vi "navX Example v2 - Dual navX.vi"() -> ()   [LabVIEW 2015]
uses:
  navX Library v2/TypeDefs/Flags/Z900_navX_Flags_OpStatusTypeDef.ctl
  navX Library v2/TypeDefs/Flags/Z900_navX_Flags_CalibrationStatusTypeDef.ctl
  navX Library v2/TypeDefs/Flags/Z900_navX_Flags_HardwareRevTypeDef.ctl
  navX Library v2/TypeDefs/Flags/Z900_navX_Flags_OmnimountConfigTypeDef.ctl
  <vilib>/Rock Robotics/SystemInterfaces/spilib/spi_bus.ctl
  NI WPI/WPI_SerialPort_USB.ctl
  navX Library v2/TypeDefs/Z900_navX_SerialStreamTypeDef.ctl
  navX Library v2/IO/Open/Z900_navX_Open_Serial.vi
  navX Library v2/IO/Open/Z900_navX_Open_SPI.vi
  navX Library v2/navX Library v2.lvlib
  NI WPI/NI WPI Serial USB.lvlib
panel:
  out "Internal error out 2":errorcluster
  out "Internal error out":errorcluster
  in  "stop":bool
  in  "Zero Yaw":bool
  out "YRPHfH 2":T1
  out "Board Information 2":T4 {"Board"."Hardware Revision" items=["navX-MXP"=33, "navX-Micro"=40]; "Omnimount Config" items=["DEFAULT", "X_UP", "X_DOWN", "Y_UP", "Y_DOWN", "Z_UP", "Z_DOWN"]}
  out "Connected 2":bool
  out "Status 2":T7 {"OP Status" items=["INITIALIZING", "SELFTEST_IN_PROGRESS", "ERROR", "IMU_AUTOCAL_IN_PROGRESS", "NORMAL"]; "Calibration Status" items=["IMU_CAL_STATE_MASK"=3, "IMU_CAL_STATE_INPROGRESS"=0, "IMU_CAL_STATE_ACCUMULATE"=1, "IMU_CAL_STATE_COMPLETE"=2]}
  out "YRPHfH":T1
  out "Board Information":T4 {"Board"."Hardware Revision" items=["navX-MXP"=33, "navX-Micro"=40]; "Omnimount Config" items=["DEFAULT", "X_UP", "X_DOWN", "Y_UP", "Y_DOWN", "Z_UP", "Z_DOWN"]}
  out "Connected":bool
  out "Status":T7 {"OP Status" items=["INITIALIZING", "SELFTEST_IN_PROGRESS", "ERROR", "IMU_AUTOCAL_IN_PROGRESS", "NORMAL"]; "Calibration Status" items=["IMU_CAL_STATE_MASK"=3, "IMU_CAL_STATE_INPROGRESS"=0, "IMU_CAL_STATE_ACCUMULATE"=1, "IMU_CAL_STATE_COMPLETE"=2]}
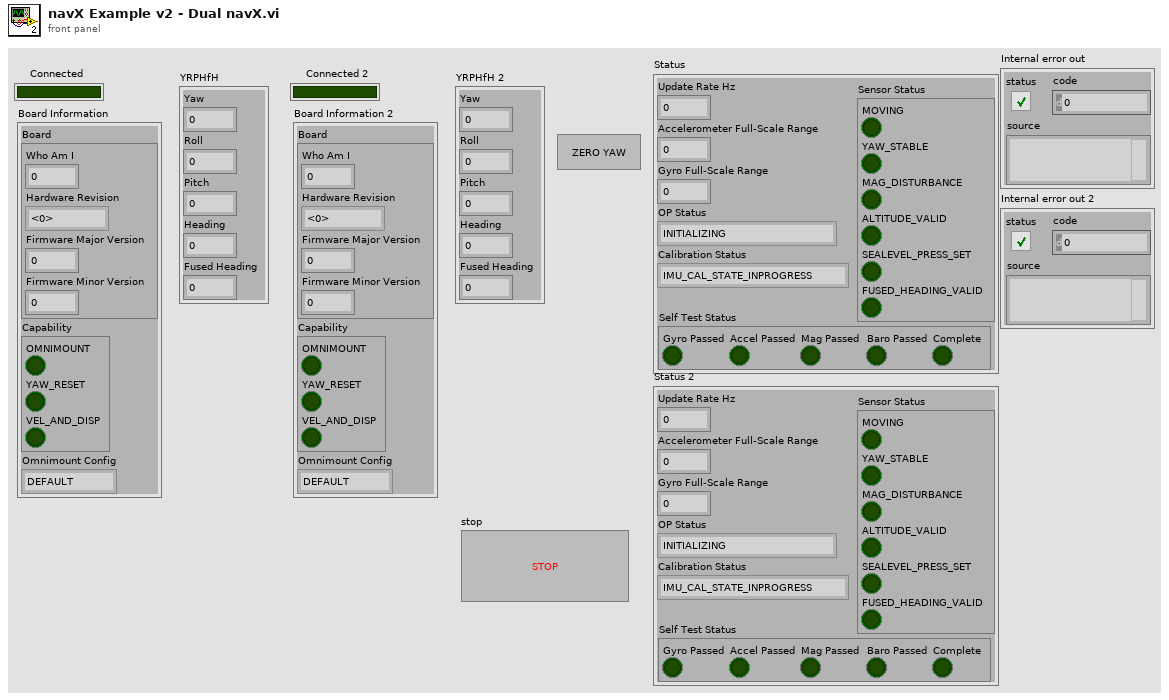
[diagram p1: front panel]
types:
  T1 = cluster{"Yaw":dbl, "Roll":dbl, "Pitch":dbl, "Heading":dbl, "Fused Heading":dbl}
  T2 = typedef "navX Library v2.lvlib/Z900_navX_Flags_HardwareRevTypeDef.ctl" = u8
  T3 = typedef "navX Library v2.lvlib/Z900_navX_Flags_OmnimountConfigTypeDef.ctl" = u8
  T4 = cluster{"Board":cluster{"Who Am I":u8, "Hardware Revision":T2, "Firmware Major Version":u8, "Firmware Minor Version":u8}, "Capability":cluster{"OMNIMOUNT":bool, "YAW_RESET":bool, "VEL_AND_DISP":bool}, "Omnimount Config":T3}
  T5 = typedef "navX Library v2.lvlib/Z900_navX_Flags_OpStatusTypeDef.ctl" = u8
  T6 = typedef "navX Library v2.lvlib/Z900_navX_Flags_CalibrationStatusTypeDef.ctl" = u8
  T7 = cluster{"Update Rate Hz":u8, "Accelerometer Full-Scale Range":u8, "Gyro Full-Scale Range":u16, "OP Status":T5, "Calibration Status":T6, "Sensor Status":cluster{"MOVING":bool, "YAW_STABLE":bool, "MAG_DISTURBANCE":bool, "ALTITUDE_VALID":bool, "SEALEVEL_PRESS_SET":bool, "FUSED_HEADING_VALID":bool}, "Self Test Status":cluster{"Gyro Passed":bool, "Accel Passed":bool, "Mag Passed":bool, "Baro Passed":bool, "Complete":bool}}
  T8 = typedef "navX Library v2.lvlib/Z900_navX_SerialStreamTypeDef.ctl" = enum16{"YRPH", "Quaterinons", "Gyro/Raw", "AHRS", "AHRSAndPositioning"}
  T9 = typedef "NI WPI Serial USB.lvlib/WPI_SerialPort_USB.ctl" = enum16{"Onboard RS-232", "MXP TTL", "USB"}
  T10 = typedef "spi_bus.ctl" = enum16{"SPI On-Board, CS0", "SPI On-Board, CS1", "SPI On-Board, CS2", "SPI On-Board, CS3", "SPI MXP", "Invalid"}
  T11 = typedef "navX Library v2.lvlib/Z900_navX_DeviceTypeDef.ctl" = cluster{"Interface":cluster{"Protocol":T12, "Update Rate (4Hz-60Hz)":u8, "navX Open TypeDef":variant}, "Notify Packet":refnum<notifier>, "Loop VI Refnum":refnum<vi>, "Ready to Close Occurrence Refnum":refnum<k4>}
  T12 = typedef "navX Library v2.lvlib/Z900_navX_ProtocolTypeDef.ctl" = enum16{"SERIAL", "I2C", "SPI"}
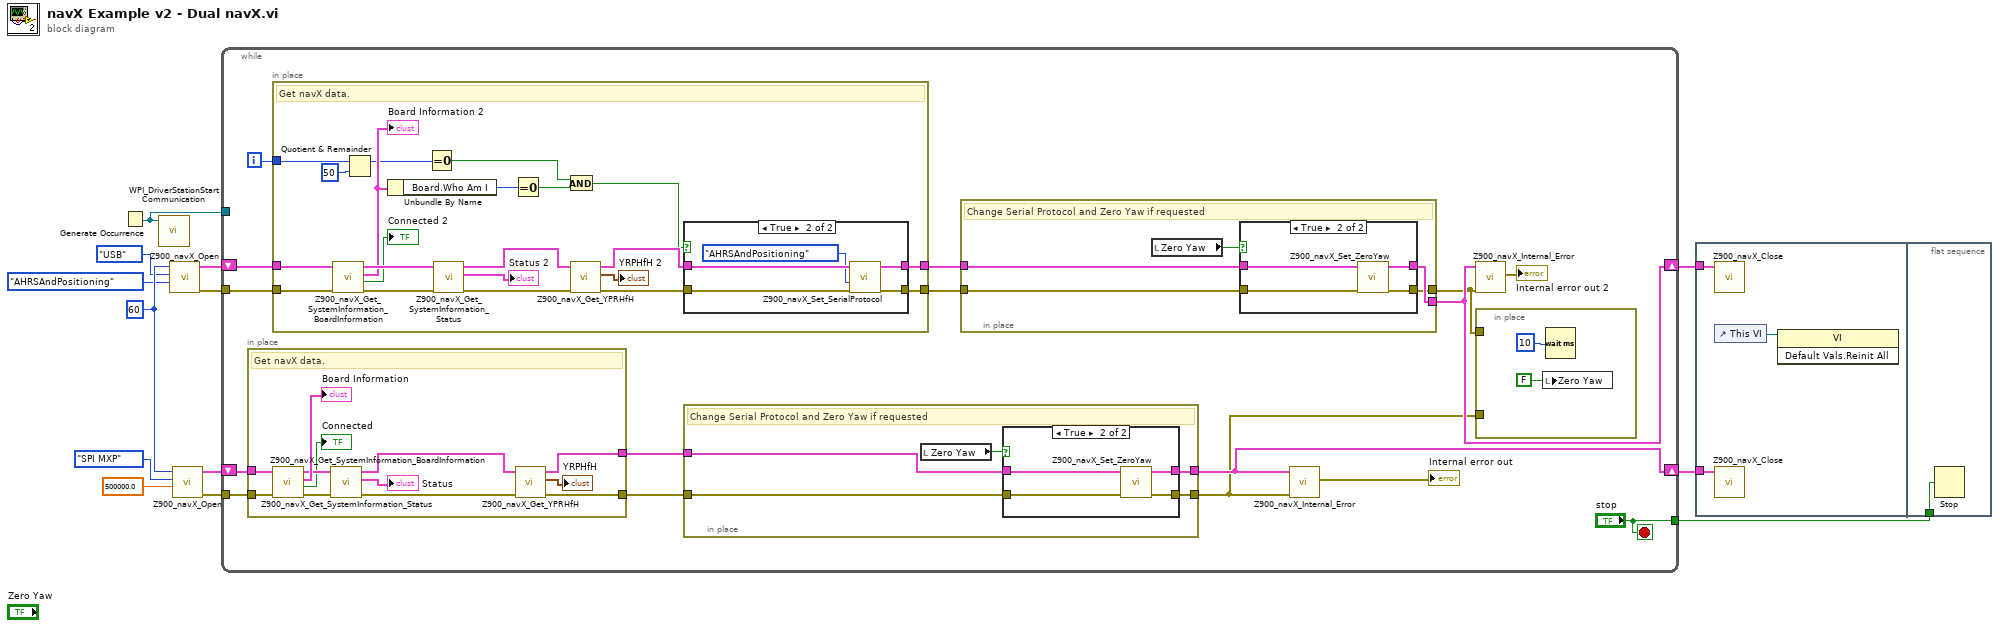
[diagram p0: block diagram]
diagram:
  w9 = u8 60 ("Update Rate (4Hz-60Hz)")
  n1 = Generate Occurrence() -> (w13:refnum<k4>)
  n2 = call <vilib>:"WPI_DriverStationStart Communication.vi"("occurrence"=w13) -> ()  [unwired: 11 in]
  n3 = call-poly "Z900_navX_Open.vi"("Stream Type"=Z900_navX_SerialStreamTypeDef."AHRSAndPositioning", "Serial Port"=WPI_SerialPort_USB."USB", "Update Rate (4Hz-60Hz)"=w9) -> ("error out"=w2:errorcluster, "navX Device"=w4:T11)  [unwired: 7 in]
  n4 = call-poly "Z900_navX_Open.vi"("Clock Rate (Hz)"=500000.0, "SPI Bus"=spi_bus."SPI MXP", "Update Rate (4Hz-60Hz)"=w9) -> ("error out"=w3:errorcluster, "navX Device"=w5:T11)  [unwired: 7 in]
  n5 = while {
    tunnel: w13 -> [_]
    shift-right: [w20] -> w11
    shift-left: w4 -> [w24]
    shift-right: [w18] -> w12
    shift-left: w5 -> [w23]
    tunnel: ["stop"] -> w10
    tunnel: w3 -> [w22]
    tunnel: w2 -> [w21]
    i -> [w14]
    stop <- "stop" stop-if-true
    n6 = in-place {
      in-place-border: [w85] -> w27
      in-place-border: [w84] -> w26
      in-place-border: w23 -> [w83]
      in-place-border: w22 -> [w82]
      # "Get navX data."
      n7 = call "Z900_navX_Get_SystemInformation_BoardInformation.vi"("error in (no error)"=w82, "navX Device"=w83) -> ("error out"=w91:errorcluster, "Connected"=→"Connected":bool, "Board Information"=→"Board Information":T4, "navX Device"=w90:T11)  [unwired: 6 in]
      n8 = call "Z900_navX_Get_SystemInformation_Status.vi"("error in (no error)"=w91, "navX Device"=w90) -> ("error out"=w86:errorcluster, "Status"=→"Status":T7, "navX Device"=w87:T11)  [unwired: 6 in, 1 out]
      n9 = call "Z900_navX_Get_YPRHfH.vi"("error in (no error)"=w86, "navX Device"=w87) -> ("error out"=w84:errorcluster, "YRPHfH"=→"YRPHfH":T1, "navX Device"=w85:T11)  [unwired: 6 in, 1 out]
    }
    n10 = in-place {
      in-place-border: [w60] -> w29
      in-place-border: [w59] -> w28
      in-place-border: w24 -> [w68]
      in-place-border: w21 -> [w67]
      in-place-border: w14 -> [w58]
      # "Get navX data."
      n11 = call "Z900_navX_Get_SystemInformation_BoardInformation.vi"("error in (no error)"=w67, "navX Device"=w68) -> ("error out"=w73:errorcluster, "Connected"=→"Connected 2":bool, "Board Information"=w65:T4, "navX Device"=w72:T11)  [unwired: 6 in]
      "Board Information 2" <- w65
      n12 = Quotient & Remainder(x=w58, y=50) -> (x-y*floor(x/y)=w56:i32)  [unwired: 1 out]
      n13 = Unbundle By Name(w65) -> ("Board.Who Am I"=w64:u8)
      n14 = Equal To 0?(x=w56) -> (x = 0?=w54:bool)
      n15 = call "Z900_navX_Get_SystemInformation_Status.vi"("error in (no error)"=w73, "navX Device"=w72) -> ("error out"=w69:errorcluster, "Status"=→"Status 2":T7, "navX Device"=w70:T11)  [unwired: 6 in, 1 out]
      n16 = Equal To 0?(x=w64) -> (x = 0?=w63:bool)
      n17 = And(x=w54, y=w63) -> (x .and. y?=w55:bool)
      n18 = call "Z900_navX_Get_YPRHfH.vi"("error in (no error)"=w69, "navX Device"=w70) -> ("error out"=w61:errorcluster, "YRPHfH"=→"YRPHfH 2":T1, "navX Device"=w62:T11)  [unwired: 6 in, 1 out]
      n19 = case shown="True" w55 {
        tunnel: w62 -> [w76 w81]
        tunnel: w61 -> [w75 w79]
        tunnel: [w76 w78] -> w60
        tunnel: [w75 w77] -> w59
        frame False {
        }
        frame True {
          n20 = call "Z900_navX_Set_SerialProtocol.vi"("error in (no error)"=w79, "Stream Type"=Z900_navX_SerialStreamTypeDef."AHRSAndPositioning", "navX Device"=w81) -> ("error out"=w77:errorcluster, "navX Device"=w78:T11)  [unwired: 7 in]
        }
      }
    }
    n21 = in-place {
      in-place-border: w27 -> [w33]
      in-place-border: w26 -> [w32]
      in-place-border: [w36] -> w18
      in-place-border: [w35] -> w17
      # "Change Serial Protocol and Zero Yaw if requested"
      n22 = local read "Zero Yaw"() -> (w34:bool)
      n23 = case shown="True" w34 {
        tunnel: w33 -> [w38 w42]
        tunnel: [w38 w41] -> w36
        tunnel: w32 -> [w37 w40]
        tunnel: [w37 w39] -> w35
        frame False {
        }
        frame True {
          n24 = call "Z900_navX_Set_ZeroYaw.vi"("error in (no error)"=w40, "navX Device"=w42) -> ("error out"=w39:errorcluster, "navX Device"=w41:T11)  [unwired: 8 in]
        }
      }
    }
    n25 = in-place {
      in-place-border: w29 -> [w44]
      in-place-border: w28 -> [w43]
      in-place-border: [w47] -> w20
      in-place-border: [w46] -> w19
      # "Change Serial Protocol and Zero Yaw if requested"
      n26 = local read "Zero Yaw"() -> (w45:bool)
      n27 = case shown="True" w45 {
        tunnel: w44 -> [w49 w53]
        tunnel: [w49 w52] -> w47
        tunnel: w43 -> [w48 w51]
        tunnel: [w48 w50] -> w46
        frame False {
        }
        frame True {
          n28 = call "Z900_navX_Set_ZeroYaw.vi"("error in (no error)"=w51, "navX Device"=w53) -> ("error out"=w50:errorcluster, "navX Device"=w52:T11)  [unwired: 8 in]
        }
      }
    }
    n29 = call "Z900_navX_Internal_Error.vi"("error in (no error)"=w17, "navX Device"=w18) -> ("Internal error out"=→"Internal error out":errorcluster)  [unwired: 7 in, 2 out]
    n30 = call "Z900_navX_Internal_Error.vi"("error in (no error)"=w19, "navX Device"=w20) -> ("Internal error out"=→"Internal error out 2":errorcluster)  [unwired: 7 in, 2 out]
    n31 = in-place {
      in-place-border: w19 -> [_]
      in-place-border: w17 -> [_]
      n32 = local write "Zero Yaw"(FALSE ("Zero Yaw")) -> ()
      n33 = Wait (ms)(milliseconds to wait=10) -> ()  [unwired: 1 out]
    }
  }
  n34 = flat-sequence {
    tunnel: w12 -> [w96]
    tunnel: w11 -> [w94]
    tunnel: w10 -> [w97]
    frame #0 {
      n35 = call "Z900_navX_Close.vi"("navX Device"=w94) -> ()  [unwired: 10 in, 1 out]
      n36 = control-ref of="This VI"() -> (w95:refnum<vi>)
      n37 = call "Z900_navX_Close.vi"("navX Device"=w96) -> ()  [unwired: 10 in, 1 out]
      n38 = invoke class="VI" method="Default Vals.Reinit All"(reference=w95) -> ()  [unwired: 2 in, 3 out]
    }
    frame #1 {
      n39 = Stop(stop? (T)=w97) -> ()
    }
  }
